vi "Get VI Version.vi"(8 "error in (no error)":errorcluster, 11 "VI in":refnum<vi>) -> (0 "error out":errorcluster, 2 "version":string, 3 "VI out":refnum<vi>)   [LabVIEW 2015]
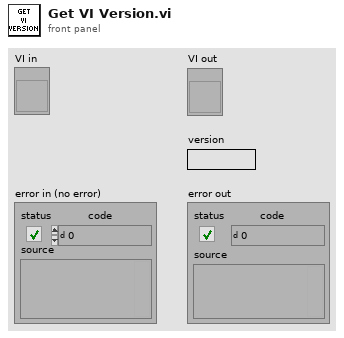
[diagram p1: front panel]
types:
  T1 = enum32{"invalid app kind", "Development System", "Run Time System", "Student Edition", "Embedded LabVIEW", "Evaluation", "Custom"}
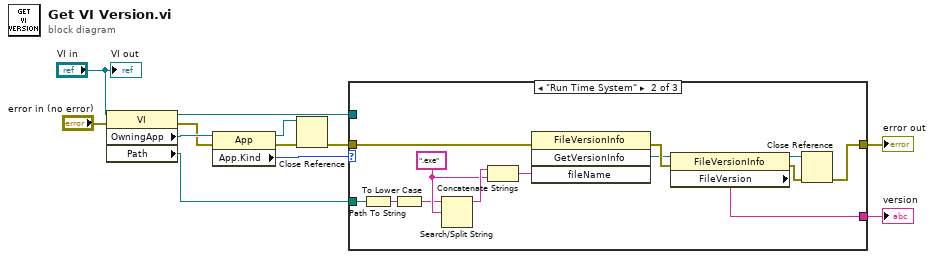
[diagram p0: block diagram]
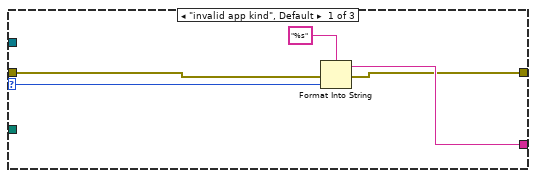
[diagram p2: hidden frame]
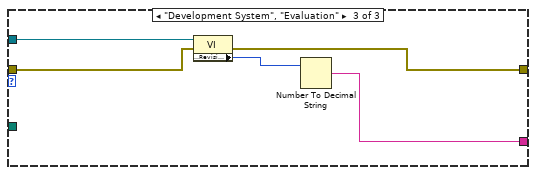
[diagram p3: hidden frame]
diagram:
  n1 = property class="VI"(reference="VI in", error in="error in (no error)") -> (reference out=w4:refnum<vi>, error out=w10:errorcluster, "OwningApp"=w11:refnum<vi>, "Path"=w1:path)
  n2 = property class="App"(reference=w11, error in=w10) -> (reference out=w8:refnum<vi>, error out=w7:errorcluster, "App.Kind"=w6:T1)
  n3 = Close Reference(reference=w8, error in (no error)=w7) -> (error out=w5:errorcluster)
  n4 = case shown="\"Run Time System\"" w6 {
    selector: w6 -> [w17 _ _]
    tunnel: [w14 w30 w31] -> w12
    tunnel: [w16 w28 w34] -> w2
    tunnel: w5 -> [w15 w24 w32]
    tunnel: w4 -> [_ _ w33]
    tunnel: w1 -> [_ w23 _]
    frame "invalid app kind", Default {
      n5 = Format Into String(format string="%s", error in=w15, w17) -> (resulting string=w16:string, error out=w14:errorcluster)  [unwired: 1 in]
    }
    frame "Run Time System" {
      w19 = ".exe" ("search string/char (-)")
      n6 = Path To String(path=w23) -> (string=w22:string)
      n7 = To Lower Case(string=w22) -> (all lower case string=w18:string)
      n8 = Search/Split String(string=w18, search string/char (-)=w19) -> (substring before match=w21:string)  [unwired: 1 in, 2 out]
      n9 = Concatenate Strings(w21, w19) -> (w20:string)
      n10 = invoke class="FileVersionInfo" method="GetVersionInfo"(error in=w24, "fileName"=w20) -> (error out=w29:errorcluster, "GetVersionInfo"=w27:refnum<k24>)  [unwired: 2 in, 2 out]
      n11 = property class="FileVersionInfo"(reference=w27, error in=w29) -> (reference out=w25:refnum<k24>, error out=w26:errorcluster, "FileVersion"=w28:string)
      n12 = Close Reference(reference=w25, error in (no error)=w26) -> (error out=w30:errorcluster)
    }
    frame "Development System", "Evaluation" {
      n13 = property class="VI"(reference=w33, error in=w32) -> (error out=w31:errorcluster, "History:Revision Number"=w35:u32)  [unwired: 1 out]
      n14 = Number To Decimal String(number=w35) -> (decimal integer string=w34:string)  [unwired: 1 in]
    }
  }
  "error out" <- w12
  "version" <- w2
  "VI out" <- "VI in"
